vi "test_SessionManagerWrapper_StopSessionManagementService_WrapperMethodsWorkWithoutError.vi"(8 "error in":errorcluster) -> (0 "error out":errorcluster, 2 "result":string, 3 "pass":bool)   [LabVIEW 2020, in "MeasurementServerTests.lvlib" / "TestStand Integration Tests.lvlib"]
uses:
  TestStand Integration Tests.lvlib
  Runtime/MeasurementLink Pin Map Client/RPC Messages/ni_measurementlink_pinmap_v1_UpdatePinMapFromXmlRequest.ctl
  Helpers/Pin Map XML Strings Global.vi
  MeasurementServerTests.lvlib
  Runtime/MeasurementLink TestStand Integration/MeasurementLink TestStand Integration.lvlib
  Runtime/MeasurementLink Pin Map Client/MeasurementLink Pin Map Client.lvlib
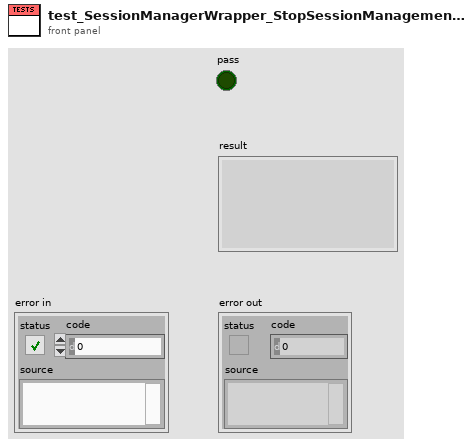
[diagram p1: front panel]
types:
  T1 = typedef "MeasurementLink Pin Map Client.lvlib/ni_measurementlink_pinmap_v1_UpdatePinMapFromXmlRequest.ctl" = cluster{"pin_map_id":string, "pin_map_xml":string}
  T2 = typedef "MeasurementLink Pin Map Client.lvlib/ni_measurementlink_pinmap_v1_PinMap.ctl" = cluster{"pin_map_id":string}
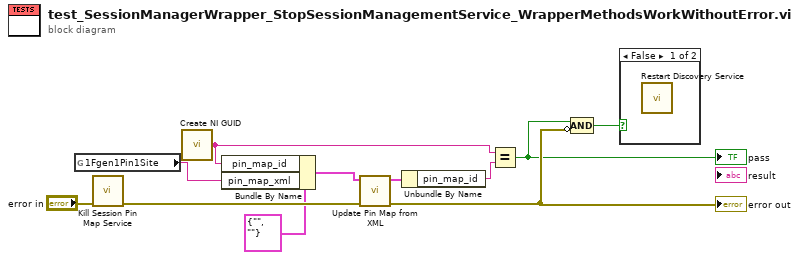
[diagram p0: block diagram]
diagram:
  n1 = global read "Pin Map XML Strings Global.vi" "1Fgen1Pin1Site"() -> (w5:string)
  n2 = call "Kill Session Pin Map Service.vi"("error in"="error in") -> ("error out"=w8:errorcluster)  [unwired: 10 in]
  n3 = call <vilib>:"Create NI GUID.vi"() -> ("NI GUID"=w4:string)
  n4 = Bundle By Name(cluster=T1 {"pin_map_id"="", "pin_map_xml"=""} ("request data"), "pin_map_id"=w4, "pin_map_xml"=w5) -> (w6:T1)
  n5 = call "Update Pin Map from XML.vi"("error in"=w8, "request data"=w6) -> ("error out"=w10:errorcluster, "response data"=w3:T2)  [unwired: 8 in]
  "error out" <- w10
  n6 = Unbundle By Name(w3) -> ("pin_map_id"=w2:string)
  n7 = Equal?(x=w4, y=w2) -> (x = y?=w1:bool)
  "pass" <- w1
  n8 = Compound Arithmetic op=AND(w1, invert w10) -> (w11:bool)
  n9 = case shown="False" w11 {
    frame False {
      n10 = call "Restart Discovery Service.vi"() -> ()  [unwired: 11 in, 1 out]
    }
    frame True {
    }
  }
